vi "TurnToAngle.vi"(8 "Error In":errorcluster, 10 "Target Angle":dbl) -> (0 "Error Out":errorcluster)   [LabVIEW 2017]
uses:
  Robot Global Data.vi
  <vilib>/addons/control/pid/pid.llb/PID (DBL).vi
  <vilib>/addons/control/pid/NI_PID_pid.lvlib
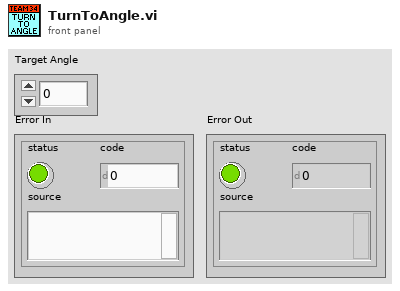
[diagram p1: front panel]
types:
  T1 = typedef "WPI_GyroDevRef.ctl" = cluster{"DevStatus":errorcluster, "Analog Channel":T2, "Gain (VoltsPerDegree/Second)":dbl, "Gyro Type":enum16{"Analog", "XRS450"}, "Handle":i32, "SPI Bus":T3, "Device Found":bool, "Sample Rate":dbl, "Calibrate On Open":bool, "Offset":dbl}
  T2 = typedef "FPGA_AIChannel.ctl" = enum8{"AI 0", "AI 1", "AI 2", "AI 3", "AI MXP 0", "AI MXP 1", "AI MXP 2", "AI MXP 3", "Invalid"}
  T3 = typedef "spi_bus.ctl" = enum16{"SPI On-Board, CS0", "SPI On-Board, CS1", "SPI On-Board, CS2", "SPI On-Board, CS3", "SPI MXP", "Invalid"}
  T4 = cluster{"proportional gain (Kc)":dbl, "integral time (Ti, min)":dbl, "derivative time (Td, min)":dbl}
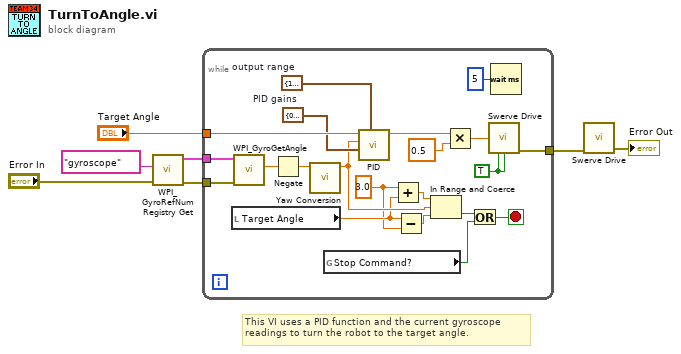
[diagram p0: block diagram]
diagram:
  # "This VI uses a PID function and the current gyroscope \nreadings to turn the robot to the target angle."
  n1 = call <vilib>:"WPI_GyroRefNum Registry Get.vi"("error in (no error)"="Error In", "refnum name"="gyroscope") -> ("error out"=w7:errorcluster, "GyroDevRef"=w6:T1)  [unwired: 8 in]
  n2 = while {
    tunnel: [w26] -> w4
    tunnel: w6 -> [w21]
    tunnel: w7 -> [w22]
    tunnel: "Target Angle" -> [w17]
    stop <- w13 stop-if-true
    w8 = 3.0 ("x")
    w15 = T4 {"proportional gain (Kc)"=0.04, "integral time (Ti, min)"=0.0, "derivative time (Td, min)"=0.0}  # PID gains
    w16 = cluster{"output high":dbl, "output low":dbl} {"output high"=1.0, "output low"=-1.0}  # output range
    w25 = TRUE ("Robot Centric?")
    n3 = local read "Target Angle"() -> (w9:dbl)
    n4 = call <vilib>:"WPI_GyroGetAngle.vi"("error in"=w22, "GyroDevRef"=w21) -> ("Angle"=w19:dbl)  [unwired: 5 in, 4 out]
    n5 = Negate(x=w19) -> (-x=w10:dbl)
    n6 = call "Yaw Conversion.vi"("Input"=w10) -> ("Output"=w11:dbl)  [unwired: 10 in]
    n7 = global read "Robot Global Data.vi" "Stop Command?"() -> (w12:bool)
    n8 = call-poly <vilib>:"PID.vi"("output range"=w16, "PID gains"=w15, "process variable"=w11, "setpoint"=w17) -> ("output"=w28:dbl)  [unwired: 6 in, 1 out]
    n9 = Add(x=w8, y=w9) -> (x+y=w24:dbl)
    n10 = Subtract(x=w9, y=w8) -> (x-y=w23:dbl)
    n11 = In Range and Coerce(upper limit=w24, x=w11, lower limit=w23) -> (In Range?=w14:bool)  [unwired: 1 out]
    n12 = Multiply(x=w28, y=0.5) -> (x*y=w20:dbl)
    n13 = Or(x=w14, y=w12) -> (x .or. y?=w13:bool)
    n14 = call "Swerve Drive.vi"("Z"=w20, "Robot Centric?"=w25, "Autonomous?"=w25) -> ("Error Out"=w26:errorcluster)  [unwired: 8 in, 4 out]
    n15 = Wait (ms)(milliseconds to wait=u32 5) -> ()  [unwired: 1 out]
  }
  n16 = call "Swerve Drive.vi"("Error In"=w4) -> ("Error Out"=→"Error Out":errorcluster)  [unwired: 10 in, 4 out]
